vi "Cluster Get Control Reference by Name.vi"(8 "error in":errorcluster, 10 "control name":string, 11 "cluster reference in":variant) -> (0 "error out":errorcluster, 1 "all control references":refnum<vi>[](array[refnum]), 2 "control reference":refnum<vi>, 3 "cluster reference out":refnum<vi>)   [LabVIEW 2020]
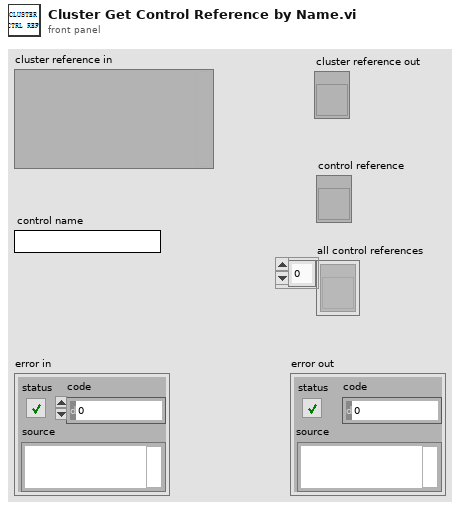
[diagram p1: front panel]
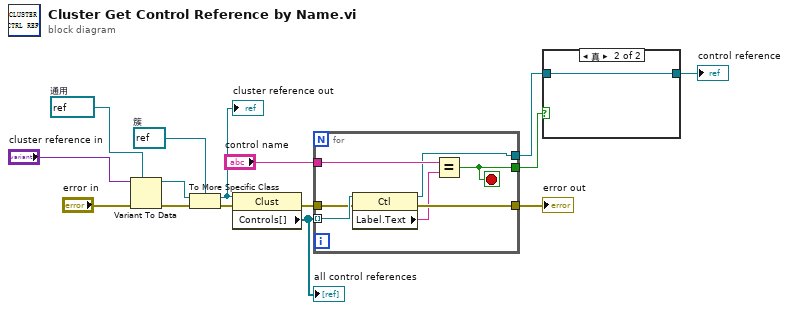
[diagram p0: block diagram]
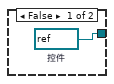
[diagram p2: hidden frame]
diagram:
  w3 = refnum<vi> refnum  # 簇
  w12 = refnum<vi> refnum  # 通用
  n1 = Variant To Data(error in="error in", type=w12, Variant="cluster reference in") -> (data=w14:refnum<vi>, error out=w2:errorcluster)
  n2 = To More Specific Class(target class=w3, reference=w14, error in=w2) -> (specific class reference=w4:refnum<vi>, error out=w1:errorcluster)
  "cluster reference out" <- w4
  n3 = property class="Clust"(reference=w4, error in=w1) -> (error out=w6:errorcluster, "Controls[]"=w13:refnum<vi>[])  [unwired: 1 out]
  "all control references" <- w13
  n4 = for {
    tunnel: w13 -> [w22] mode=indexing
    tunnel: "control name" -> [w21]
    tunnel: [w20] -> w10
    tunnel: [w19] -> w9
    tunnel: w6 -> [w18]
    tunnel: [w17] -> w5
    stop <- w20 stop-if-true
    n5 = property class="Ctl"(reference=w22, error in=w18) -> (reference out=w19:refnum<vi>, error out=w17:errorcluster, "Label.Text"=w16:string)
    n6 = Equal?(x=w21, y=w16) -> (x = y?=w20:bool)
  }
  "error out" <- w5
  n7 = case shown="真" w10 {
    tunnel: w9 -> [_ w24]
    tunnel: [w23 w24] -> w8
    frame False {
      w23 = refnum<vi> refnum  # 控件
    }
    frame True {
    }
  }
  "control reference" <- w8
